vi "Instrument Perform Autorange.vi"(0 "Session In":refnum<visa-resource-name>="GPIB0::16::INSTR", 7 "error in":errorcluster {"code" format="%.0x"}, 11 "Perform AutoRange":bool) -> (20 "Session Out":refnum<visa-resource-name>, 27 "error out":errorcluster {"code" format="%.0x"})   [LabVIEW 2018]
doc: "Launches the Instrument I/O Assistant, which you can use to communicate with message-based instruments and graphically parse the response. For example you can communicate with an instrument that uses a serial, Ethernet, or GPIB interface."
panel:
  in  "Timeout":u32=3000
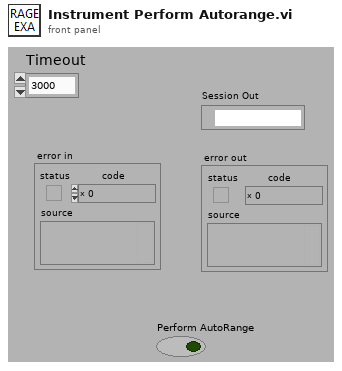
[diagram p1: front panel]
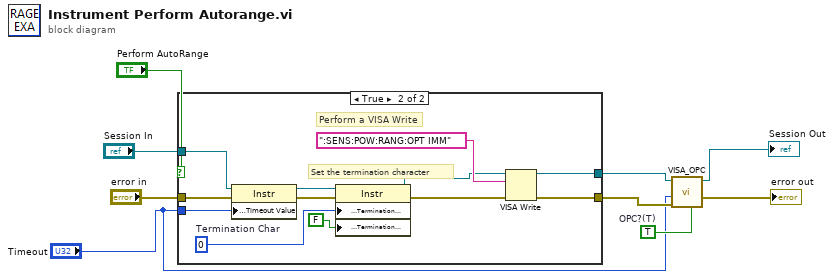
[diagram p0: block diagram]
diagram:
  w2 = TRUE  # OPC?(T)
  n1 = case shown="True" "Perform AutoRange" {
    tunnel: "error in" -> [w10 w23]
    tunnel: "Session In" -> [w11 w22]
    tunnel: [w10 w16] -> w7
    tunnel: [w11 w13] -> w4
    tunnel: "Timeout" -> [_ w12]
    frame False {
    }
    frame True {
      w19 = u8 0  # Termination Char
      # "Perform a VISA Write"
      # "Set the termination character"
      n2 = property class="Instr"(reference=w22, error in=w23, "General Settings:Timeout Value"=w12) -> (reference out=w18:refnum<visa-resource-name>, error out=w21:errorcluster)
      n3 = property class="Instr"(reference=w18, error in=w21, "Message Based Settings:Termination Character"=w19, "Message Based Settings:Termination Character Enable"=FALSE ("enable")) -> (reference out=w14:refnum<visa-resource-name>, error out=w20:errorcluster)
      n4 = VISA Write(VISA resource name=w14, write buffer=":SENS:POW:RANG:OPT IMM" ("StaticText"), error in (no error)=w20) -> (VISA resource name out=w13:refnum<visa-resource-name>, error out=w16:errorcluster)  [unwired: 1 out]
    }
  }
  n5 = call "VISA_OPC.vi"("OPC(T)"=w2, "error in"=w7, "Timeout"="Timeout", "Session In"=w4) -> ("error out"=→"error out":errorcluster, "Session Out"=→"Session Out":refnum<visa-resource-name>)  [unwired: 5 in, 1 out]
